vi "dynamic lqr.vi"() -> ()   [LabVIEW 2016]
panel:
  out "lambda actual":dbl
  out "omega_actual":dbl
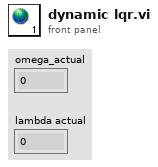
[diagram p1: front panel]
diagram:
